vi "App - analyze RUS V6.vi"() -> ()   [LabVIEW 2015] (continued)
"Norm  Ampl"=0.023595886932381915, "z (inf)"=0.19378474353100264-0.42084593191813147i, "4corners"={"z (-pi/2)"=-0.40484593191813145-0.16978474353100262i, "z(inf)"=0.19378474353100264-0.42084593191813147i, "z (pi/2)"=0.4448459319181315+0.17778474353100263i, "z center"=0.020000000000000018+0.0040000000000000036i, "z(0)"=-0.1537847435310026+0.4288459319181315i, "radius"=0.45901547136400744}}, "timestamp(min)"=551.5166666656733, "timestamp"=timestamp(3493760912 s since 1904-01-01), "Magn Field(T)"=0.0}, {"temperature"=107.207, "lorentzian"={"Amplitude"=0.00019486220005198642, "omega(0)"=667.9206130476543, "Gamma"=0.050419907186881614, "phase"=3.5490376394277394, "Q"=13247.160701268322, "Norm  Ampl"=0.023216607976607278, "z (inf)"=0.20246610113930197-0.41876972105888066i, "4corners"={"z (-pi/2)"=-0.40276972105888065-0.17846610113930195i, "z(inf)"=0.20246610113930197-0.41876972105888066i, "z (pi/2)"=0.4427697210588807+0.18646610113930195i, "z center"=0.020000000000000018+0.0040000000000000036i, "z(0)"=-0.16246610113930193+0.42676972105888067i, "radius"=0.46046510737425234}}, "timestamp(min)"=552.8500000014901, "timestamp"=timestamp(3493760992 s since 1904-01-01), "Magn Field(T)"=0.0}, {"temperature"=107.004, "lorentzian"={"Amplitude"=0.00020084030643088081, "omega(0)"=667.9097751474013, "Gamma"=0.051914717697569265, "phase"=3.5402670225649624, "Q"=12865.518773276002, "Norm  Ampl"=0.023856106137013743, "z (inf)"=0.1983861988709874-0.4194873195080103i, "4corners"={"z (-pi/2)"=-0.4034873195080103-0.17438619887098739i, "z(inf)"=0.1983861988709874-0.4194873195080103i, "z (pi/2)"=0.44348731950801035+0.1823861988709874i, "z center"=0.020000000000000018+0.0040000000000000036i, "z(0)"=-0.15838619887098737+0.42748731950801033i, "radius"=0.45952491306970406}}, "timestamp(min)"=554.1666666641831, "timestamp"=timestamp(3493761071 s since 1904-01-01), "Magn Field(T)"=0.0}, {"temperature"=106.803, "lorentzian"={"Amplitude"=0.00020210598584422863, "omega(0)"=667.9032383407135, "Gamma"=0.0519377350819643, "phase"=3.5458751895017375, "Q"=12859.691268529094, "Norm  Ampl"=0.023961487843567296, "z (inf)"=0.2014763877931069-0.42015844644330047i, "4corners"={"z (-pi/2)"=-0.40415844644330046-0.17747638779310687i, "z(inf)"=0.2014763877931069-0.42015844644330047i, "z (pi/2)"=0.4441584464433005+0.18547638779310688i, "z center"=0.020000000000000018+0.0040000000000000036i, "z(0)"=-0.16147638779310686+0.4281584464433005i, "radius"=0.46135026500006293}}, "timestamp(min)"=555.4833333343267, "timestamp"=timestamp(3493761150 s since 1904-01-01), "Magn Field(T)"=0.0}, {"temperature"=106.609, "lorentzian"={"Amplitude"=0.00020717135714785185, "omega(0)"=667.900021351503, "Gamma"=0.05268344288947372, "phase"=3.586329553478829, "Q"=12677.607702152492, "Norm  Ampl"=0.024204953723853912, "z (inf)"=0.21766104912826675-0.4107487090456408i, "4corners"={"z (-pi/2)"=-0.3947487090456408-0.19366104912826673i, "z(inf)"=0.21766104912826675-0.4107487090456408i, "z (pi/2)"=0.43474870904564084+0.20166104912826674i, "z center"=0.020000000000000018+0.0040000000000000036i, "z(0)"=-0.17766104912826672+0.4187487090456408i, "radius"=0.45944138037132953}}, "timestamp(min)"=556.8166666701436, "timestamp"=timestamp(3493761230 s since 1904-01-01), "Magn Field(T)"=0.0}, {"temperature"=106.409, "lorentzian"={"Amplitude"=0.0002048000866120398, "omega(0)"=667.8939948673919, "Gamma"=0.05168289309927176, "phase"=3.5792743045660185, "Q"=12922.921973127757, "Norm  Ampl"=0.02374217561013892, "z (inf)"=0.21470470623045562-0.4120788739011124i, "4corners"={"z (-pi/2)"=-0.3960788739011124-0.1907047062304556i, "z(inf)"=0.21470470623045562-0.4120788739011124i, "z (pi/2)"=0.43607887390111244+0.1987047062304556i, "z center"=0.020000000000000018+0.0040000000000000036i, "z(0)"=-0.1747047062304556+0.4200788739011124i, "radius"=0.4593817061389208}}, "timestamp(min)"=558.1333333328366, "timestamp"=timestamp(3493761309 s since 1904-01-01), "Magn Field(T)"=0.0}, {"temperature"=106.218, "lorentzian"={"Amplitude"=0.00025572189236614705, "omega(0)"=667.8857574673999, "Gamma"=0.06129103331630066, "phase"=3.5613155843645803, "Q"=10896.957047871672, "Norm  Ampl"=0.029834403901466296, "z (inf)"=0.2983608556677271-0.45651581823489573i, "4corners"={"z (-pi/2)"=-0.34451581823489574-0.21036085566772708i, "z(inf)"=0.2983608556677271-0.45651581823489573i, "z (pi/2)"=0.5445158182348957+0.18636085566772706i, "z center"=0.09999999999999998-0.01200000000000001i, "z(0)"=-0.09836085566772709+0.4325158182348957i, "radius"=0.48676620848439317}}, "timestamp(min)"=559.4666666686535, "timestamp"=timestamp(3493761389 s since 1904-01-01), "Magn Field(T)"=0.0}, {"temperature"=106.019, "lorentzian"={"Amplitude"=0.0002632435711688871, "omega(0)"=667.8761489000353, "Gamma"=0.06224234569653387, "phase"=3.514320252965729, "Q"=10730.253518341096, "Norm  Ampl"=0.031031630855244, "z (inf)"=0.28155467225607145-0.48432894382839947i, "4corners"={"z (-pi/2)"=-0.3643289438283995-0.20155467225607146i, "z(inf)"=0.28155467225607145-0.48432894382839947i, "z (pi/2)"=0.5643289438283994+0.16155467225607142i, "z center"=0.09999999999999998-0.020000000000000018i, "z(0)"=-0.08155467225607146+0.44432894382839944i, "radius"=0.4985613975177044}}, "timestamp(min)"=560.7833333313465, "timestamp"=timestamp(3493761468 s since 1904-01-01), "Magn Field(T)"=0.0}, {"temperature"=105.822, "lorentzian"={"Amplitude"=0.0002684955921345172, "omega(0)"=667.873197176711, "Gamma"=0.06457346286091041, "phase"=3.5701517127628164, "Q"=10342.843136898091, "Norm  Ampl"=0.03185297785375564, "z (inf)"=0.3049888938507378-0.4686730026378616i, "4corners"={"z (-pi/2)"=-0.3486730026378616-0.22498889385073786i, "z(inf)"=0.3049888938507378-0.4686730026378616i, "z (pi/2)"=0.5486730026378616+0.18498889385073783i, "z center"=0.09999999999999998-0.020000000000000018i, "z(0)"=-0.10498889385073787+0.42867300263786157i, "radius"=0.49328278897425926}}, "timestamp(min)"=562.1000000014901, "timestamp"=timestamp(3493761547 s since 1904-01-01), "Magn Field(T)"=0.0}, {"temperature"=105.631, "lorentzian"={"Amplitude"=0.00021658869264008107, "omega(0)"=667.8687353967621, "Gamma"=0.05339114257672214, "phase"=3.6070003340669543, "Q"=12508.980013623916, "Norm  Ampl"=0.024817091513203788, "z (inf)"=0.2206037388767987-0.41137812798398815i, "4corners"={"z (-pi/2)"=-0.40337812798398814-0.2046037388767987i, "z(inf)"=0.2206037388767987-0.41137812798398815i, "z (pi/2)"=0.42737812798398817+0.2126037388767987i, "z center"=0.01200000000000001+0.0040000000000000036i, "z(0)"=-0.1966037388767987+0.41937812798398816i, "radius"=0.46481664027965053}}, "timestamp(min)"=563.433333337307, "timestamp"=timestamp(3493761627 s since 1904-01-01), "Magn Field(T)"=0.0}, {"temperature"=105.436, "lorentzian"={"Amplitude"=0.0002218314180916303, "omega(0)"=667.8714445455947, "Gamma"=0.054199629091694894, "phase"=3.6696044505572583, "Q"=12322.435701832761, "Norm  Ampl"=0.025127965694294544, "z (inf)"=0.2455789779506424-0.39647875154155293i, "4corners"={"z (-pi/2)"=-0.3884787515415529-0.2295789779506424i, "z(inf)"=0.2455789779506424-0.39647875154155293i, "z (pi/2)"=0.41247875154155295+0.2375789779506424i, "z center"=0.01200000000000001+0.0040000000000000036i, "z(0)"=-0.22157897795064238+0.40447875154155294i, "radius"=0.46361877591049694}}, "timestamp(min)"=564.75, "timestamp"=timestamp(3493761706 s since 1904-01-01), "Magn Field(T)"=0.0}, {"temperature"=105.248, "lorentzian"={"Amplitude"=0.000227469417377074, "omega(0)"=667.8742869887905, "Gamma"=0.055611282796684904, "phase"=3.7311880764042153, "Q"=12009.690361406369, "Norm  Ampl"=0.025864391335479804, "z (inf)"=0.27060297115865334-0.38256894611561193i, "4corners"={"z (-pi/2)"=-0.3745689461156119-0.2546029711586533i, "z(inf)"=0.27060297115865334-0.38256894611561193i, "z (pi/2)"=0.39856894611561194+0.26260297115865333i, "z center"=0.01200000000000001+0.0040000000000000036i, "z(0)"=-0.24660297115865332+0.39056894611561194i, "radius"=0.4650925142302531}}, "timestamp(min)"=566.0666666701436, "timestamp"=timestamp(3493761785 s since 1904-01-01), "Magn Field(T)"=0.0}, {"temperature"=105.052, "lorentzian"={"Amplitude"=0.0002429700925118724, "omega(0)"=667.8871818169091, "Gamma"=0.060003132898738556, "phase"=3.8580015567320327, "Q"=11130.871832043124, "Norm  Ampl"=0.027880260178402085, "z (inf)"=0.317124509739482-0.3464220710794713i, "4corners"={"z (-pi/2)"=-0.3384220710794713-0.30112450973948196i, "z(inf)"=0.317124509739482-0.3464220710794713i, "z (pi/2)"=0.36242207107947133+0.30912450973948197i, "z center"=0.01200000000000001+0.0040000000000000036i, "z(0)"=-0.29312450973948195+0.3544220710794713i, "radius"=0.4646467414535318}}, "timestamp(min)"=567.3999999985099, "timestamp"=timestamp(3493761865 s since 1904-01-01), "Magn Field(T)"=0.0}, {"temperature"=104.861, "lorentzian"={"Amplitude"=0.0002502763365307906, "omega(0)"=667.8929742135593, "Gamma"=0.06019253835777101, "phase"=3.873429728997418, "Q"=11095.942992863213, "Norm  Ampl"=0.028276910251888523, "z (inf)"=0.32592081029646364-0.34548771027033914i, "4corners"={"z (-pi/2)"=-0.33748771027033914-0.3099208102964636i, "z(inf)"=0.32592081029646364-0.34548771027033914i, "z (pi/2)"=0.36148771027033916+0.31792081029646363i, "z center"=0.01200000000000001+0.0040000000000000036i, "z(0)"=-0.3019208102964636+0.35348771027033915i, "radius"=0.4697743445178683}}, "timestamp(min)"=568.7166666686535, "timestamp"=timestamp(3493761944 s since 1904-01-01), "Magn Field(T)"=0.0}, {"temperature"=104.676, "lorentzian"={"Amplitude"=0.0002521607020805991, "omega(0)"=667.8950769727215, "Gamma"=0.060407263727030744, "phase"=3.8571373884805884, "Q"=11056.535849576236, "Norm  Ampl"=0.028597788222530274, "z (inf)"=0.3225747074308711-0.3533043822481044i, "4corners"={"z (-pi/2)"=-0.3453043822481044-0.30657470743087106i, "z(inf)"=0.3225747074308711-0.3533043822481044i, "z (pi/2)"=0.3693043822481044+0.31457470743087107i, "z center"=0.01200000000000001+0.0040000000000000036i, "z(0)"=-0.29857470743087106+0.3613043822481044i, "radius"=0.4734163817079745}}, "timestamp(min)"=570.0500000044703, "timestamp"=timestamp(3493762024 s since 1904-01-01), "Magn Field(T)"=0.0}, {"temperature"=104.483, "lorentzian"={"Amplitude"=0.0002616699298388773, "omega(0)"=667.9087317249022, "Gamma"=0.06096226834913139, "phase"=3.9202466618051206, "Q"=10956.10038490995, "Norm  Ampl"=0.029379986156093177, "z (inf)"=0.35047506364287284-0.33907158972615603i, "4corners"={"z (-pi/2)"=-0.331071589726156-0.3344750636428728i, "z(inf)"=0.35047506364287284-0.33907158972615603i, "z (pi/2)"=0.35507158972615604+0.34247506364287283i, "z center"=0.01200000000000001+0.0040000000000000036i, "z(0)"=-0.3264750636428728+0.34707158972615604i, "radius"=0.48193722037759107}}, "timestamp(min)"=571.3666666671634, "timestamp"=timestamp(3493762103 s since 1904-01-01), "Magn Field(T)"=0.0}, {"temperature"=104.301, "lorentzian"={"Amplitude"=0.0002561983592771509, "omega(0)"=667.9127020137031, "Gamma"=0.060621059428511107, "phase"=3.8340778636883632, "Q"=11017.832883659115, "Norm  Ampl"=0.028653015315670247, "z (inf)"=0.313769267945375-0.3597865927431585i, "4corners"={"z (-pi/2)"=-0.3517865927431585-0.297769267945375i, "z(inf)"=0.313769267945375-0.3597865927431585i, "z (pi/2)"=0.3757865927431585+0.305769267945375i, "z center"=0.01200000000000001+0.0040000000000000036i, "z(0)"=-0.289769267945375+0.3677865927431585i, "radius"=0.47265777909176976}}, "timestamp(min)"=572.683333337307, "timestamp"=timestamp(3493762182 s since 1904-01-01), "Magn Field(T)"=0.0}, {"temperature"=104.111, "lorentzian"={"Amplitude"=0.0002696422038201607, "omega(0)"=667.9290862382628, "Gamma"=0.06200781003801521, "phase"=3.865091187068677, "Q"=10771.692885602226, "Norm  Ampl"=0.029165667218756523, "z (inf)"=0.32337993905547086-0.3485281729508489i, "4corners"={"z (-pi/2)"=-0.3405281729508489-0.30737993905547084i, "z(inf)"=0.32337993905547086-0.3485281729508489i, "z (pi/2)"=0.36452817295084894+0.31537993905547085i, "z center"=0.01200000000000001+0.0040000000000000036i, "z(0)"=-0.29937993905547083+0.35652817295084893i, "radius"=0.47035473758669893}}, "timestamp(min)"=574.0166666656733, "timestamp"=timestamp(3493762262 s since 1904-01-01), "Magn Field(T)"=0.0}, {"temperature"=103.923, "lorentzian"={"Amplitude"=0.0003015863280613358, "omega(0)"=667.9424835071507, "Gamma"=0.06499393815641434, "phase"=3.906968159973645, "Q"=10276.996631588641, "Norm  Ampl"=0.03086802283868664, "z (inf)"=0.34104004021284723-0.338487605050504i, "4corners"={"z (-pi/2)"=-0.330487605050504-0.3250400402128472i, "z(inf)"=0.34104004021284723-0.338487605050504i, "z (pi/2)"=0.35448760505050403+0.3330400402128472i, "z center"=0.01200000000000001+0.0040000000000000036i, "z(0)"=-0.3170400402128472+0.346487605050504i, "radius"=0.47493695126458857}}, "timestamp(min)"=575.3333333358169, "timestamp"=timestamp(3493762341 s since 1904-01-01), "Magn Field(T)"=0.0}, {"temperature"=103.741, "lorentzian"={"Amplitude"=0.00028572502145804223, "omega(0)"=667.9529480751149, "Gamma"=0.06065156532371923, "phase"=3.8694852502487116, "Q"=11012.954810152214, "Norm  Ampl"=0.02841886421040113, "z (inf)"=0.3237315596025237-0.3458162300361338i, "4corners"={"z (-pi/2)"=-0.3378162300361338-0.3077315596025237i, "z(inf)"=0.3237315596025237-0.3458162300361338i, "z (pi/2)"=0.36181623003613383+0.3157315596025237i, "z center"=0.01200000000000001+0.0040000000000000036i, "z(0)"=-0.2997315596025237+0.3538162300361338i, "radius"=0.4685594519897289}}, "timestamp(min)"=576.6499999985099, "timestamp"=timestamp(3493762420 s since 1904-01-01), "Magn Field(T)"=0.0}, {"temperature"=103.554, "lorentzian"={"Amplitude"=0.00029347828497651077, "omega(0)"=667.9649600314765, "Gamma"=0.0606160090228989, "phase"=3.879604993693491, "Q"=11019.612983413992, "Norm  Ampl"=0.0281993037467068, "z (inf)"=0.32500345866369346-0.3401673681453368i, "4corners"={"z (-pi/2)"=-0.3321673681453368-0.30900345866369344i, "z(inf)"=0.32500345866369346-0.3401673681453368i, "z (pi/2)"=0.35616736814533684+0.31700345866369345i, "z center"=0.01200000000000001+0.0040000000000000036i, "z(0)"=-0.30100345866369344+0.34816736814533683i, "radius"=0.46521214776865216}}, "timestamp(min)"=577.9833333343267, "timestamp"=timestamp(3493762500 s since 1904-01-01), "Magn Field(T)"=0.0}, {"temperature"=103.375, "lorentzian"={"Amplitude"=0.00029593239910138665, "omega(0)"=667.9769292525697, "Gamma"=0.06010812192011819, "phase"=3.835573129918802, "Q"=11112.922978034318, "Norm  Ampl"=0.028010585074310118, "z (inf)"=0.31005668992413643-0.3542196458950623i, "4corners"={"z (-pi/2)"=-0.34621964589506227-0.2940566899241364i, "z(inf)"=0.31005668992413643-0.3542196458950623i, "z (pi/2)"=0.3702196458950623+0.3020566899241364i, "z center"=0.01200000000000001+0.0040000000000000036i, "z(0)"=-0.2860566899241364+0.3622196458950623i, "radius"=0.4660033316551681}}, "timestamp(min)"=579.3000000044703, "timestamp"=timestamp(3493762579 s since 1904-01-01), "Magn Field(T)"=0.0}, {"temperature"=103.189, "lorentzian"={"Amplitude"=0.0003024991177126299, "omega(0)"=667.9949531202576, "Gamma"=0.061445029051674135, "phase"=3.8802215177408033, "Q"=10871.423830860038, "Norm  Ampl"=0.028605256156809217, "z (inf)"=0.3254378260432909-0.34021839261030223i, "4corners"={"z (-pi/2)"=-0.3322183926103022-0.3094378260432909i, "z(inf)"=0.3254378260432909-0.34021839261030223i, "z (pi/2)"=0.35621839261030225+0.3174378260432909i, "z center"=0.01200000000000001+0.0040000000000000036i, "z(0)"=-0.3014378260432909+0.34821839261030224i, "radius"=0.46554223503992037}}, "timestamp(min)"=580.6333333328366, "timestamp"=timestamp(3493762659 s since 1904-01-01), "Magn Field(T)"=0.0}, {"temperature"=103.003, "lorentzian"={"Amplitude"=0.0003034545800900397, "omega(0)"=668.0129403654028, "Gamma"=0.06109581920259991, "phase"=3.92974403360385, "Q"=10933.85683478937, "Norm  Ampl"=0.02856607938524639, "z (inf)"=0.3435252179875782-0.32570470417851566i, "4corners"={"z (-pi/2)"=-0.31770470417851565-0.32752521798757817i, "z(inf)"=0.3435252179875782-0.32570470417851566i, "z (pi/2)"=0.3417047041785157+0.3355252179875782i, "z center"=0.01200000000000001+0.0040000000000000036i, "z(0)"=-0.31952521798757816+0.33370470417851567i, "radius"=0.4675619339928709}}, "timestamp(min)"=581.9500000029802, "timestamp"=timestamp(3493762738 s since 1904-01-01), "Magn Field(T)"=0.0}, {"temperature"=102.827, "lorentzian"={"Amplitude"=0.0003082226354358521, "omega(0)"=668.0268805358065, "Gamma"=0.061379010302154334, "phase"=3.9369231608328588, "Q"=10883.637211601626, "Norm  Ampl"=0.028528456303629258, "z (inf)"=0.3439054565307153-0.3213768875994757i, "4corners"={"z (-pi/2)"=-0.3133768875994757-0.3279054565307153i, "z(inf)"=0.3439054565307153-0.3213768875994757i, "z (pi/2)"=0.3373768875994757+0.3359054565307153i, "z center"=0.01200000000000001+0.0040000000000000036i, "z(0)"=-0.3199054565307153+0.3293768875994757i, "radius"=0.4647917286901568}}, "timestamp(min)"=583.2666666656733, "timestamp"=timestamp(3493762817 s since 1904-01-01), "Magn Field(T)"=0.0}, {"temperature"=102.644, "lorentzian"={"Amplitude"=0.0003053588931030111, "omega(0)"=668.0419170256847, "Gamma"=0.05967413478657053, "phase"=3.9137884253488755, "Q"=11194.832056048937, "Norm  Ampl"=0.02775934410541557, "z (inf)"=0.3285622248733565-0.3292473896508297i, "4corners"={"z (-pi/2)"=-0.3292473896508297-0.3205622248733565i, "z(inf)"=0.3285622248733565-0.3292473896508297i, "z (pi/2)"=0.33724738965082973+0.3285622248733565i, "z center"=0.0040000000000000036+0.0040000000000000036i, "z(0)"=-0.3205622248733565+0.33724738965082973i, "radius"=0.465182179929364}}, "timestamp(min)"=584.6000000014901, "timestamp"=timestamp(3493762897 s since 1904-01-01), "Magn Field(T)"=0.0}, {"temperature"=102.47, "lorentzian"={"Amplitude"=0.00029264692102488155, "omega(0)"=668.0495978156077, "Gamma"=0.0595853414327936, "phase"=3.820280053328173, "Q"=11211.643363143297, "Norm  Ampl"=0.027175229932189106, "z (inf)"=0.2983094126795748-0.34300557493473105i, "4corners"={"z (-pi/2)"=-0.34300557493473105-0.27430941267957476i, "z(inf)"=0.2983094126795748-0.34300557493473105i, "z (pi/2)"=0.36700557493473107+0.2983094126795748i, "z center"=0.01200000000000001+0.01200000000000001i, "z(0)"=-0.27430941267957476+0.36700557493473107i, "radius"=0.4560724043654275}}, "timestamp(min)"=585.9166666641831, "timestamp"=timestamp(3493762976 s since 1904-01-01), "Magn Field(T)"=0.0}, {"temperature"=102.285, "lorentzian"={"Amplitude"=0.0003025643445775688, "omega(0)"=668.0649496135221, "Gamma"=0.06070963041109803, "phase"=3.8061005148865608, "Q"=11004.266458051052, "Norm  Ampl"=0.028236166919451102, "z (inf)"=0.29081524431594935-0.3621377210977686i, "4corners"={"z (-pi/2)"=-0.3621377210977686-0.28281524431594934i, "z(inf)"=0.29081524431594935-0.3621377210977686i, "z (pi/2)"=0.3701377210977686+0.29081524431594935i, "z center"=0.0040000000000000036+0.0040000000000000036i, "z(0)"=-0.28281524431594934+0.3701377210977686i, "radius"=0.46510194063526017}}, "timestamp(min)"=587.2333333343267, "timestamp"=timestamp(3493763055 s since 1904-01-01), "Magn Field(T)"=0.0}, {"temperature"=102.107, "lorentzian"={"Amplitude"=0.0003040535108698859, "omega(0)"=668.0806226434124, "Gamma"=0.06115547204039357, "phase"=3.854607343006187, "Q"=10924.29835554439, "Norm  Ampl"=0.02837099766505297, "z (inf)"=0.3074553105550051-0.3469029271504728i, "4corners"={"z (-pi/2)"=-0.3469029271504728-0.29945531055500507i, "z(inf)"=0.3074553105550051-0.3469029271504728i, "z (pi/2)"=0.3549029271504728+0.3074553105550051i, "z center"=0.0040000000000000036+0.0040000000000000036i, "z(0)"=-0.29945531055500507+0.3549029271504728i, "radius"=0.4639159296540749}}, "timestamp(min)"=588.5666666701436, "timestamp"=timestamp(3493763135 s since 1904-01-01), "Magn Field(T)"=0.0}, {"temperature"=101.933, "lorentzian"={"Amplitude"=0.0003045292994418805, "omega(0)"=668.0882919601835, "Gamma"=0.060089684248189376, "phase"=3.8334688630900136, "Q"=11118.186096647934, "Norm  Ampl"=0.027630599395966043, "z (inf)"=0.2973590869823717-0.35008662671530094i, "4corners"={"z (-pi/2)"=-0.35008662671530094-0.28935908698237167i, "z(inf)"=0.2973590869823717-0.35008662671530094i, "z (pi/2)"=0.35808662671530095+0.2973590869823717i, "z center"=0.0040000000000000036+0.0040000000000000036i, "z(0)"=-0.28935908698237167+0.35808662671530095i, "radius"=0.45982267574984986}}, "timestamp(min)"=589.8833333328366, "timestamp"=timestamp(3493763214 s since 1904-01-01), "Magn Field(T)"=0.0}, {"temperature"=101.753, "lorentzian"={"Amplitude"=0.0003037710470755072, "omega(0)"=668.0896160369514, "Gamma"=0.05972007259123305, "phase"=3.7477522031773276, "Q"=11187.019490244682, "Norm  Ampl"=0.02735290558813929, "z (inf)"=0.26494027642095813-0.37241896051065276i, "4corners"={"z (-pi/2)"=-0.37241896051065276-0.2569402764209581i, "z(inf)"=0.26494027642095813-0.37241896051065276i, "z (pi/2)"=0.38041896051065277+0.26494027642095813i, "z center"=0.0040000000000000036+0.0040000000000000036i, "z(0)"=-0.2569402764209581+0.38041896051065277i, "radius"=0.45801862592100595}}, "timestamp(min)"=591.2166666686535, "timestamp"=timestamp(3493763294 s since 1904-01-01), "Magn Field(T)"=0.0}, {"temperature"=101.581, "lorentzian"={"Amplitude"=0.000302078866754409, "omega(0)"=668.0963848127388, "Gamma"=0.0599802045144248, "phase"=3.7558698597649096, "Q"=11138.614651640053, "Norm  Ampl"=0.02747965264494422, "z (inf)"=0.2600603331756243-0.37039192729720777i, "4corners"={"z (-pi/2)"=-0.3783919272972078-0.2600603331756243i, "z(inf)"=0.2600603331756243-0.37039192729720777i, "z (pi/2)"=0.37039192729720777+0.26806033317562433i, "z center"=-0.0040000000000000036+0.0040000000000000036i, "z(0)"=-0.26806033317562433+0.3783919272972078i, "radius"=0.4581453642482257}}, "timestamp(min)"=592.5333333313465, "timestamp"=timestamp(3493763373 s since 1904-01-01), "Magn Field(T)"=0.0}, {"temperature"=101.405, "lorentzian"={"Amplitude"=0.0003108565243422264, "omega(0)"=668.0981322511478, "Gamma"=0.061828381286781205, "phase"=3.7099961266104287, "Q"=10805.686940958067, "Norm  Ampl"=0.028443989485532707, "z (inf)"=0.24363767688032925-0.38371025554489496i, "4corners"={"z (-pi/2)"=-0.39171025554489497-0.24363767688032925i, "z(inf)"=0.24363767688032925-0.38371025554489496i, "z (pi/2)"=0.38371025554489496+0.25163767688032923i, "z center"=-0.0040000000000000036+0.0040000000000000036i, "z(0)"=-0.25163767688032923+0.39171025554489497i, "radius"=0.4600474554492983}}, "timestamp(min)"=593.8500000014901, "timestamp"=timestamp(3493763452 s since 1904-01-01), "Magn Field(T)"=0.0}, {"temperature"=101.228, "lorentzian"={"Amplitude"=0.0003020301382464617, "omega(0)"=668.106726291208, "Gamma"=0.06020689263535034, "phase"=3.7709860286183976, "Q"=11096.847836636742, "Norm  Ampl"=0.027857329782784164, "z (inf)"=0.2603665224546951-0.37003426042319687i, "4corners"={"z (-pi/2)"=-0.3860342604231969-0.2683665224546951i, "z(inf)"=0.2603665224546951-0.37003426042319687i, "z (pi/2)"=0.36203426042319686+0.2763665224546951i, "z center"=-0.01200000000000001+0.0040000000000000036i, "z(0)"=-0.2843665224546951+0.3780342604231969i, "radius"=0.4626933655504386}}, "timestamp(min)"=595.183333337307, "timestamp"=timestamp(3493763532 s since 1904-01-01), "Magn Field(T)"=0.0}, {"temperature"=101.06, "lorentzian"={"Amplitude"=0.00030380203856116456, "omega(0)"=668.1148687330386, "Gamma"=0.062304287256802524, "phase"=3.994129183908156, "Q"=10723.417250232524, "Norm  Ampl"=0.028895346092586947, "z (inf)"=0.32920245687613864-0.3092007602601433i, "4corners"={"z (-pi/2)"=-0.32520076026014333-0.35320245687613866i, "z(inf)"=0.32920245687613864-0.3092007602601433i, "z (pi/2)"=0.2852007602601433+0.34520245687613865i, "z center"=-0.020000000000000018-0.0040000000000000036i, "z(0)"=-0.3692024568761387+0.3012007602601433i, "radius"=0.4637778131300601}}, "timestamp(min)"=596.5, "timestamp"=timestamp(3493763611 s since 1904-01-01), "Magn Field(T)"=0.0}, {"temperature"=100.883, "lorentzian"={"Amplitude"=0.00031274625965722327, "omega(0)"=668.1099013064036, "Gamma"=0.061377185457406856, "phase"=4.034131725545669, "Q"=10885.313432464955, "Norm  Ampl"=0.02837201159282308, "z (inf)"=0.33194415997419624-0.29403690108049374i, "4corners"={"z (-pi/2)"=-0.31803690108049376-0.36394415997419627i, "z(inf)"=0.33194415997419624-0.29403690108049374i, "z (pi/2)"=0.2620369010804937+0.35594415997419626i, "z center"=-0.028000000000000025-0.0040000000000000036i, "z(0)"=-0.3879441599741963+0.28603690108049373i, "radius"=0.4622566411506771}}, "timestamp(min)"=597.8166666701436, "timestamp"=timestamp(3493763690 s since 1904-01-01), "Magn Field(T)"=0.0}, {"temperature"=100.708, "lorentzian"={"Amplitude"=0.00032983716903870185, "omega(0)"=668.1117303235795, "Gamma"=0.06337015040226514, "phase"=3.997894082453735, "Q"=10543.003702571268, "Norm  Ampl"=0.029125538556145768, "z (inf)"=0.3272003679195827-0.30515281935840516i, "4corners"={"z (-pi/2)"=-0.3211528193584052-0.3512003679195827i, "z(inf)"=0.3272003679195827-0.30515281935840516i, "z (pi/2)"=0.28115281935840514+0.3432003679195827i, "z center"=-0.020000000000000018-0.0040000000000000036i, "z(0)"=-0.3672003679195827+0.29715281935840515i, "radius"=0.45960974325073856}}, "timestamp(min)"=599.1499999985099, "timestamp"=timestamp(3493763770 s since 1904-01-01), "Magn Field(T)"=0.0}, {"temperature"=100.542, "lorentzian"={"Amplitude"=0.0003375908707174886, "omega(0)"=668.1110147726321, "Gamma"=0.06296077379815741, "phase"=4.004675687295234, "Q"=10611.543894210918, "Norm  Ampl"=0.02903392790328897, "z (inf)"=0.330399807670561-0.3037881841743976i, "4corners"={"z (-pi/2)"=-0.31978818417439764-0.354399807670561i, "z(inf)"=0.330399807670561-0.3037881841743976i, "z (pi/2)"=0.2797881841743976+0.346399807670561i, "z center"=-0.020000000000000018-0.0040000000000000036i, "z(0)"=-0.370399807670561+0.2957881841743976i, "radius"=0.4611431237545982}}, "timestamp(min)"=600.4666666686535, "timestamp"=timestamp(3493763849 s since 1904-01-01), "Magn Field(T)"=0.0}, {"temperature"=100.369, "lorentzian"={"Amplitude"=0.0003550013944215624, "omega(0)"=668.1116377961806, "Gamma"=0.06477225965592939, "phase"=4.042901482522946, "Q"=10314.78045300864, "Norm  Ampl"=0.029936374392811195, "z (inf)"=0.3424129116351151-0.2908209463291375i, "4corners"={"z (-pi/2)"=-0.30682094632913753-0.36641291163511513i, "z(inf)"=0.3424129116351151-0.2908209463291375i, "z (pi/2)"=0.2668209463291375+0.35841291163511513i, "z center"=-0.020000000000000018-0.0040000000000000036i, "z(0)"=-0.38241291163511515+0.2828209463291375i, "radius"=0.46217894129112347}}, "timestamp(min)"=601.8000000044703, "timestamp"=timestamp(3493763929 s since 1904-01-01), "Magn Field(T)"=0.0}, {"temperature"=100.203, "lorentzian"={"Amplitude"=0.0003706837977447706, "omega(0)"=668.1101255100197, "Gamma"=0.06572611819726708, "phase"=4.060268465318725, "Q"=10165.062897899848, "Norm  Ampl"=0.030250199261476044, "z (inf)"=0.34580312045882133-0.2833110906831418i, "4corners"={"z (-pi/2)"=-0.2993110906831418-0.36980312045882135i, "z(inf)"=0.34580312045882133-0.2833110906831418i, "z (pi/2)"=0.2593110906831418+0.36180312045882135i, "z center"=-0.020000000000000018-0.0040000000000000036i, "z(0)"=-0.38580312045882137+0.2753110906831418i, "radius"=0.4602462474763018}}, "timestamp(min)"=603.1166666671634, "timestamp"=timestamp(3493764008 s since 1904-01-01), "Magn Field(T)"=0.0}, {"temperature"=100.032, "lorentzian"={"Amplitude"=0.00037967247624858837, "omega(0)"=668.1053232498274, "Gamma"=0.06584499571993843, "phase"=3.9991489781466187, "Q"=10146.637811193894, "Norm  Ampl"=0.030400743328454584, "z (inf)"=0.32916000767855236-0.306085592008112i, "4corners"={"z (-pi/2)"=-0.322085592008112-0.3531600076785524i, "z(inf)"=0.32916000767855236-0.306085592008112i, "z (pi/2)"=0.28208559200811195+0.34516000767855237i, "z center"=-0.020000000000000018-0.0040000000000000036i, "z(0)"=-0.3691600076785524+0.29808559200811197i, "radius"=0.4617016524347495}}, "timestamp(min)"=604.433333337307, "timestamp"=timestamp(3493764087 s since 1904-01-01), "Magn Field(T)"=0.0}, {"temperature"=99.859, "lorentzian"={"Amplitude"=0.00038782950008322653, "omega(0)"=668.1031913806788, "Gamma"=0.06644204729174678, "phase"=3.978004083416531, "Q"=10055.427528399903, "Norm  Ampl"=0.030410619471739425, "z (inf)"=0.3197257186357181-0.3107197858801527i, "4corners"={"z (-pi/2)"=-0.3267197858801527-0.3437257186357181i, "z(inf)"=0.3197257186357181-0.3107197858801527i, "z (pi/2)"=0.2867197858801527+0.3357257186357181i, "z center"=-0.020000000000000018-0.0040000000000000036i, "z(0)"=-0.3597257186357181+0.3027197858801527i, "radius"=0.4577014211829824}}, "timestamp(min)"=605.7666666656733, "timestamp"=timestamp(3493764167 s since 1904-01-01), "Magn Field(T)"=0.0}, {"temperature"=99.697, "lorentzian"={"Amplitude"=0.0004044492174666845, "omega(0)"=668.1004691432302, "Gamma"=0.06745889627707242, "phase"=3.938290307625674, "Q"=9903.81559756264, "Norm  Ampl"=0.030952952100896446, "z (inf)"=0.30809538073647513-0.32476329613897237i, "4corners"={"z (-pi/2)"=-0.3407632961389724-0.33209538073647515i, "z(inf)"=0.30809538073647513-0.32476329613897237i, "z (pi/2)"=0.30076329613897235+0.32409538073647515i, "z center"=-0.020000000000000018-0.0040000000000000036i, "z(0)"=-0.34809538073647517+0.31676329613897236i, "radius"=0.45884166224368805}}, "timestamp(min)"=607.0833333358169, "timestamp"=timestamp(3493764246 s since 1904-01-01), "Magn Field(T)"=0.0}, {"temperature"=99.53, "lorentzian"={"Amplitude"=0.000410169349517558, "omega(0)"=668.0992433152304, "Gamma"=0.06816978956278076, "phase"=3.9024939864198034, "Q"=9800.51790683535, "Norm  Ampl"=0.0315119027256548, "z (inf)"=0.30676002832077287-0.3307727123087024i, "4corners"={"z (-pi/2)"=-0.34677271230870244-0.3147600283207729i, "z(inf)"=0.30676002832077287-0.3307727123087024i, "z (pi/2)"=0.3227727123087024+0.3227600283207729i, "z center"=-0.01200000000000001+0.0040000000000000036i, "z(0)"=-0.3307600283207729+0.33877271230870243i, "radius"=0.4622561244176059}}, "timestamp(min)"=608.3999999985099, "timestamp"=timestamp(3493764325 s since 1904-01-01), "Magn Field(T)"=0.0}, {"temperature"=99.368, "lorentzian"={"Amplitude"=0.0003957792315444673, "omega(0)"=668.1003509236078, "Gamma"=0.06515472917129171, "phase"=3.8417781433153624, "Q"=10254.05767810304, "Norm  Ampl"=0.02969968455467861, "z (inf)"=0.281720433112044-0.3445859370169715i, "4corners"={"z (-pi/2)"=-0.3605859370169715-0.289720433112044i, "z(inf)"=0.281720433112044-0.3445859370169715i, "z (pi/2)"=0.3365859370169715+0.297720433112044i, "z center"=-0.01200000000000001+0.0040000000000000036i, "z(0)"=-0.305720433112044+0.3525859370169715i, "radius"=0.4558331364803646}}, "timestamp(min)"=609.7333333343267, "timestamp"=timestamp(3493764405 s since 1904-01-01), "Magn Field(T)"=0.0}, {"temperature"=99.199, "lorentzian"={"Amplitude"=0.00037984684163067155, "omega(0)"=668.1064053025405, "Gamma"=0.0640270896309424, "phase"=3.84342904967562, "Q"=10434.7458107742, "Norm  Ampl"=0.02971642632268455, "z (inf)"=0.28764743903678774-0.35043095488121356i, "4corners"={"z (-pi/2)"=-0.3664309548812136-0.29564743903678775i, "z(inf)"=0.28764743903678774-0.35043095488121356i, "z (pi/2)"=0.34243095488121356+0.30364743903678776i, "z center"=-0.01200000000000001+0.0040000000000000036i, "z(0)"=-0.31164743903678777+0.35843095488121357i, "radius"=0.464122709527679}}, "timestamp(min)"=611.0500000044703, "timestamp"=timestamp(3493764484 s since 1904-01-01), "Magn Field(T)"=0.0}, {"temperature"=99.032, "lorentzian"={"Amplitude"=0.0003802727618714869, "omega(0)"=668.1052302227044, "Gamma"=0.06439691099622996, "phase"=3.7986953222412385, "Q"=10374.802453829157, "Norm  Ampl"=0.029664693950564147, "z (inf)"=0.2773791630516989-0.3607298513702428i, "4corners"={"z (-pi/2)"=-0.36872985137024283-0.2773791630516989i, "z(inf)"=0.2773791630516989-0.3607298513702428i, "z (pi/2)"=0.3607298513702428+0.2853791630516989i, "z center"=-0.0040000000000000036+0.0040000000000000036i, "z(0)"=-0.2853791630516989+0.36872985137024283i, "radius"=0.46065398932412815}}, "timestamp(min)"=612.3833333328366, "timestamp"=timestamp(3493764564 s since 1904-01-01), "Magn Field(T)"=0.0}, {"temperature"=98.874, "lorentzian"={"Amplitude"=0.0003732423860535719, "omega(0)"=668.1022726722371, "Gamma"=0.06270428830253441, "phase"=3.692928630467542, "Q"=10654.80991425643, "Norm  Ampl"=0.028773799510568566, "z (inf)"=0.23637360944953553-0.3868864252447063i, "4corners"={"z (-pi/2)"=-0.3948864252447063-0.23637360944953553i, "z(inf)"=0.23637360944953553-0.3868864252447063i, "z (pi/2)"=0.3868864252447063+0.24437360944953554i, "z center"=-0.0040000000000000036+0.0040000000000000036i, "z(0)"=-0.24437360944953554+0.3948864252447063i, "radius"=0.4588808882056249}}, "timestamp(min)"=613.7000000029802, "timestamp"=timestamp(3493764643 s since 1904-01-01), "Magn Field(T)"=0.0}, {"temperature"=98.708, "lorentzian"={"Amplitude"=0.0003773753970576512, "omega(0)"=668.1004679566593, "Gamma"=0.06260911490376811, "phase"=3.6913687888681883, "Q"=10670.977684056828, "Norm  Ampl"=0.028961151595897867, "z (inf)"=0.2376915888003912-0.390407110240003i, "4corners"={"z (-pi/2)"=-0.398407110240003-0.2376915888003912i, "z(inf)"=0.2376915888003912-0.390407110240003i, "z (pi/2)"=0.390407110240003+0.24569158880039121i, "z center"=-0.0040000000000000036+0.0040000000000000036i, "z(0)"=-0.24569158880039121+0.398407110240003i, "radius"=0.46257085155111893}}, "timestamp(min)"=615.0166666656733, "timestamp"=timestamp(3493764722 s since 1904-01-01), "Magn Field(T)"=0.0}, {"temperature"=98.551, "lorentzian"={"Amplitude"=0.000377856329112072, "omega(0)"=668.0972424835554, "Gamma"=0.062134740416682814, "phase"=3.620400580913716, "Q"=10752.394522021295, "Norm  Ampl"=0.028766106178541542, "z (inf)"=0.2092971518890126-0.40690067855140216i, "4corners"={"z (-pi/2)"=-0.41490067855140217-0.2092971518890126i, "z(inf)"=0.2092971518890126-0.40690067855140216i, "z (pi/2)"=0.40690067855140216+0.2172971518890126i, "z center"=-0.0040000000000000036+0.0040000000000000036i, "z(0)"=-0.2172971518890126+0.41490067855140217i, "radius"=0.4629633275303426}}, "timestamp(min)"=616.3500000014901, "timestamp"=timestamp(3493764802 s since 1904-01-01), "Magn Field(T)"=0.0}, {"temperature"=98.387, "lorentzian"={"Amplitude"=0.0003938897630412544, "omega(0)"=668.0965315443399, "Gamma"=0.06519188458261926, "phase"=3.644171514236587, "Q"=10248.154901821328, "Norm  Ampl"=0.030190698860140756, "z (inf)"=0.21907178915620049-0.4018391015265461i, "4corners"={"z (-pi/2)"=-0.4098391015265461-0.21907178915620049i, "z(inf)"=0.21907178915620049-0.4018391015265461i, "z (pi/2)"=0.4018391015265461+0.2270717891562005i, "z center"=-0.0040000000000000036+0.0040000000000000036i, "z(0)"=-0.2270717891562005+0.4098391015265461i, "radius"=0.4631051710413333}}, "timestamp(min)"=617.6666666641831, "timestamp"=timestamp(3493764881 s since 1904-01-01), "Magn Field(T)"=0.0}, {"temperature"=98.223, "lorentzian"={"Amplitude"=0.0003756643243931179, "omega(0)"=668.0939847231178, "Gamma"=0.06130583961108929, "phase"=3.643374665980686, "Q"=10897.721798793697, "Norm  Ampl"=0.028451021233058163, "z (inf)"=0.21921883336987233-0.40287434867102817i, "4corners"={"z (-pi/2)"=-0.4108743486710282-0.21921883336987233i, "z(inf)"=0.21921883336987233-0.40287434867102817i, "z (pi/2)"=0.40287434867102817+0.22721883336987234i, "z center"=-0.0040000000000000036+0.0040000000000000036i, "z(0)"=-0.22721883336987234+0.4108743486710282i, "radius"=0.4640833795531577}}, "timestamp(min)"=618.9833333343267, "timestamp"=timestamp(3493764960 s since 1904-01-01), "Magn Field(T)"=0.0}, {"temperature"=98.065, "lorentzian"={"Amplitude"=0.0004042234382466762, "omega(0)"=668.0907103744488, "Gamma"=0.06544516539130649, "phase"=3.657982507258787, "Q"=10208.404339416578, "Norm  Ampl"=0.030144749408719033, "z (inf)"=0.23142379257796578-0.39655052054112405i, "4corners"={"z (-pi/2)"=-0.39655052054112405-0.22342379257796577i, "z(inf)"=0.23142379257796578-0.39655052054112405i, "z (pi/2)"=0.40455052054112406+0.23142379257796578i, "z center"=0.0040000000000000036+0.0040000000000000036i, "z(0)"=-0.22342379257796577+0.40455052054112406i, "radius"=0.4606107911635495}}, "timestamp(min)"=620.3166666701436, "timestamp"=timestamp(3493765040 s since 1904-01-01), "Magn Field(T)"=0.0}, {"temperature"=97.905, "lorentzian"={"Amplitude"=0.0004042853296374257, "omega(0)"=668.0884812262261, "Gamma"=0.06540919413204768, "phase"=3.6395966663942216, "Q"=10213.984289081642, "Norm  Ampl"=0.03027439392740258, "z (inf)"=0.21708908361214796-0.4026278140981054i, "4corners"={"z (-pi/2)"=-0.4106278140981054-0.21708908361214796i, "z(inf)"=0.21708908361214796-0.4026278140981054i, "z (pi/2)"=0.4026278140981054+0.22508908361214797i, "z center"=-0.0040000000000000036+0.0040000000000000036i, "z(0)"=-0.22508908361214797+0.4106278140981054i, "radius"=0.4628461538034671}}, "timestamp(min)"=621.6333333328366, "timestamp"=timestamp(3493765119 s since 1904-01-01), "Magn Field(T)"=0.0}, {"temperature"=97.749, "lorentzian"={"Amplitude"=0.0004087269810925043, "omega(0)"=668.0853168502122, "Gamma"=0.0663465240202537, "phase"=3.65400400929897, "Q"=10069.63554935093, "Norm  Ampl"=0.03076333547229797, "z (inf)"=0.22333154863665175-0.4001242672403644i, "4corners"={"z (-pi/2)"=-0.4081242672403644-0.22333154863665175i, "z(inf)"=0.22333154863665175-0.4001242672403644i, "z (pi/2)"=0.4001242672403644+0.23133154863665176i, "z center"=-0.0040000000000000036+0.0040000000000000036i, "z(0)"=-0.23133154863665176+0.4081242672403644i, "radius"=0.46367667223842496}}, "timestamp(min)"=622.9666666686535, "timestamp"=timestamp(3493765199 s since 1904-01-01), "Magn Field(T)"=0.0}, {"temperature"=97.59, "lorentzian"={"Amplitude"=0.00039188163918809515, "omega(0)"=668.0833849424677, "Gamma"=0.06536266839707777, "phase"=3.705874177452739, "Q"=10221.176725586929, "Norm  Ampl"=0.030482327990007087, "z (inf)"=0.24541177458432759-0.3900589753860805i, "4corners"={"z (-pi/2)"=-0.3980589753860805-0.24541177458432759i, "z(inf)"=0.24541177458432759-0.3900589753860805i, "z (pi/2)"=0.3900589753860805+0.2534117745843276i, "z center"=-0.0040000000000000036+0.0040000000000000036i, "z(0)"=-0.2534117745843276+0.3980589753860805i, "radius"=0.4663568476860086}}, "timestamp(min)"=624.2833333313465, "timestamp"=timestamp(3493765278 s since 1904-01-01), "Magn Field(T)"=0.0}, {"temperature"=97.43, "lorentzian"={"Amplitude"=0.00038566369757841865, "omega(0)"=668.0812319431826, "Gamma"=0.06381512149640996, "phase"=3.716070712362109, "Q"=10469.01136090083, "Norm  Ampl"=0.029837120217934353, "z (inf)"=0.2500681974663812-0.3885017593872999i, "4corners"={"z (-pi/2)"=-0.3965017593872999-0.2500681974663812i, "z(inf)"=0.2500681974663812-0.3885017593872999i, "z (pi/2)"=0.3885017593872999+0.2580681974663812i, "z center"=-0.0040000000000000036+0.0040000000000000036i, "z(0)"=-0.2580681974663812+0.3965017593872999i, "radius"=0.4675556438392568}}, "timestamp(min)"=625.6000000014901, "timestamp"=timestamp(3493765357 s since 1904-01-01), "Magn Field(T)"=0.0}, {"temperature"=97.276, "lorentzian"={"Amplitude"=0.0003857015903030322, "omega(0)"=668.076925264809, "Gamma"=0.0633548437111985, "phase"=3.730951896880218, "Q"=10545.001552055299, "Norm  Ampl"=0.029643450345640737, "z (inf)"=0.25606967929819635-0.38496017912631714i, "4corners"={"z (-pi/2)"=-0.39296017912631714-0.25606967929819635i, "z(inf)"=0.25606967929819635-0.38496017912631714i, "z (pi/2)"=0.38496017912631714+0.26406967929819636i, "z center"=-0.0040000000000000036+0.0040000000000000036i, "z(0)"=-0.26406967929819636+0.39296017912631714i, "radius"=0.4678955642408286}}, "timestamp(min)"=626.933333337307, "timestamp"=timestamp(3493765437 s since 1904-01-01), "Magn Field(T)"=0.0}, {"temperature"=97.118, "lorentzian"={"Amplitude"=0.00039543609597437345, "omega(0)"=668.0728404783213, "Gamma"=0.06585116299399046, "phase"=3.7327646024563776, "Q"=10145.194254796825, "Norm  Ampl"=0.030621135992630222, "z (inf)"=0.24716344580206806-0.38208831058364484i, "4corners"={"z (-pi/2)"=-0.39808831058364486-0.25516344580206807i, "z(inf)"=0.24716344580206806-0.38208831058364484i, "z (pi/2)"=0.37408831058364483+0.2631634458020681i, "z center"=-0.01200000000000001+0.0040000000000000036i, 
